vi "Kickforce.vi"(8 "AI Parameters":T1={"GotoKick"={"Dist do cone a frente"=150.0, "attacker farback"=1500.0, "Perto"=300.0, "min dist to kick"=150.0, "kick eps"=0.05, "Time to transition"=0.0}, "Attacker"={"CC chute"=0.09, "CC passe"=0.045, "Kick Force"=100.0, "ball-robot Kick"=200.0, "ball-robot Pass"=0.3, "drible\nAttk"=FALSE}, "Defender"={"D max"=1700.0, "Vel p/ robô av"=1000.0, "Kick Force"=100.0, "D atk-def"=0.0, "D farback"=0.0, "drible\ndef"=FALSE, "drible\ngoalie"=FALSE}, "Timeout"={"Field/v in x"=6.0, "Dist Robots"=300, "Dist up in y"=300}, "Pose Striker"={"dist"=200.0, "Numeric"=-4.0, "dist 2"=200.0, "drible\nstriker"=FALSE}, "Dist Stop"=300.0, "D ball out"=200, "D central gap "=150.0, "T pass"=0.0, "Force ++"=0.0, "range kick"=0.0, "Chute alto"=TRUE, "Marcador novo"=TRUE, "drible"=FALSE, "D drible"=300.0} {"D drible" format="%#_13g"; "D central gap" format="%#_13g"; "Dist Stop" format="%#_13g"; "Pose Striker"."Numeric" format="%#_13g"; "Defender"."Kick Force" format="%#_13g"; "Defender"."Vel p/ robô av" format="%#_13g"; "Attacker"."ball-robot Kick" format="%#_13g"; "Attacker"."Kick Force" format="%#_13g"; "Attacker"."CC passe" format="%#_13g"; "Attacker"."CC chute" format="%#_13g"; "GotoKick"."kick eps" format="%#_13g"; "GotoKick"."min dist to kick" format="%#_13g"; "GotoKick"."Perto" format="%#_13g"; "GotoKick"."attacker farback" format="%#_13g"; "GotoKick"."Dist do cone a frente" format="%#_13g"}, 10 "Distância ao\nalvo do chute":dbl=1.23 format="%#_13g") -> (1 "Tempo até  bola\nchegar ao alvo":dbl, 2 "Força do chute":dbl)   [LabVIEW 2017]
uses:
  AI Parameters.ctl
panel:
  in  "y":dbl=12.0
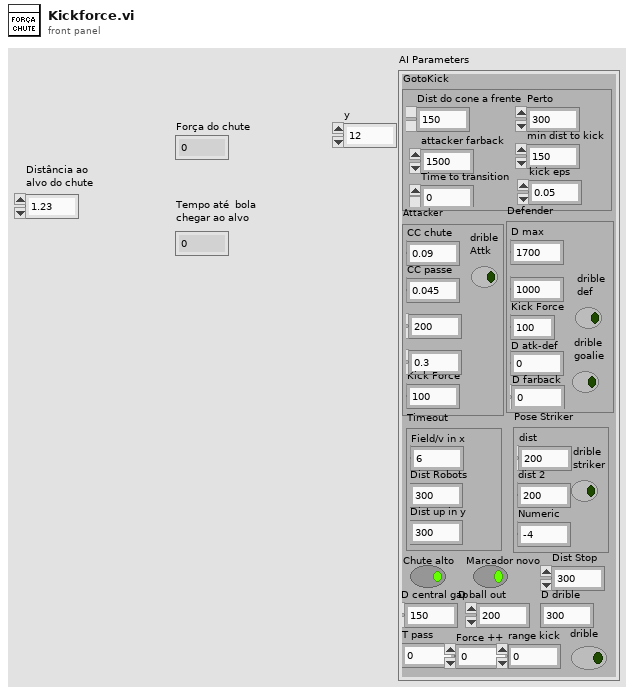
[diagram p1: front panel]
types:
  T1 = typedef "AI Parameters.ctl" = cluster{"GotoKick":cluster{"Dist do cone a frente":dbl, "attacker farback":dbl, "Perto":dbl, "min dist to kick":dbl, "kick eps":dbl, "Time to transition":dbl}, "Attacker":cluster{"CC chute":dbl, "CC passe":dbl, "Kick Force":dbl, "ball-robot Kick":dbl, "ball-robot Pass":dbl, "drible\nAttk":bool}, "Defender":cluster{"D max":dbl, "Vel p/ robô av":dbl, "Kick Force":dbl, "D atk-def":dbl, "D farback":dbl, "drible\ndef":bool, "drible\ngoalie":bool}, "Timeout":cluster{"Field/v in x":dbl, "Dist Robots":u32, "Dist up in y":u32}, "Pose Striker":cluster{"dist":dbl, "Numeric":dbl, "dist 2":dbl, "drible\nstriker":bool}, "Dist Stop":dbl, "D ball out":i32, "D central gap ":dbl, "T pass":dbl, "Force ++":dbl, "range kick":dbl, "Chute alto":bool, "Marcador novo":bool, "drible":bool, "D drible":dbl}
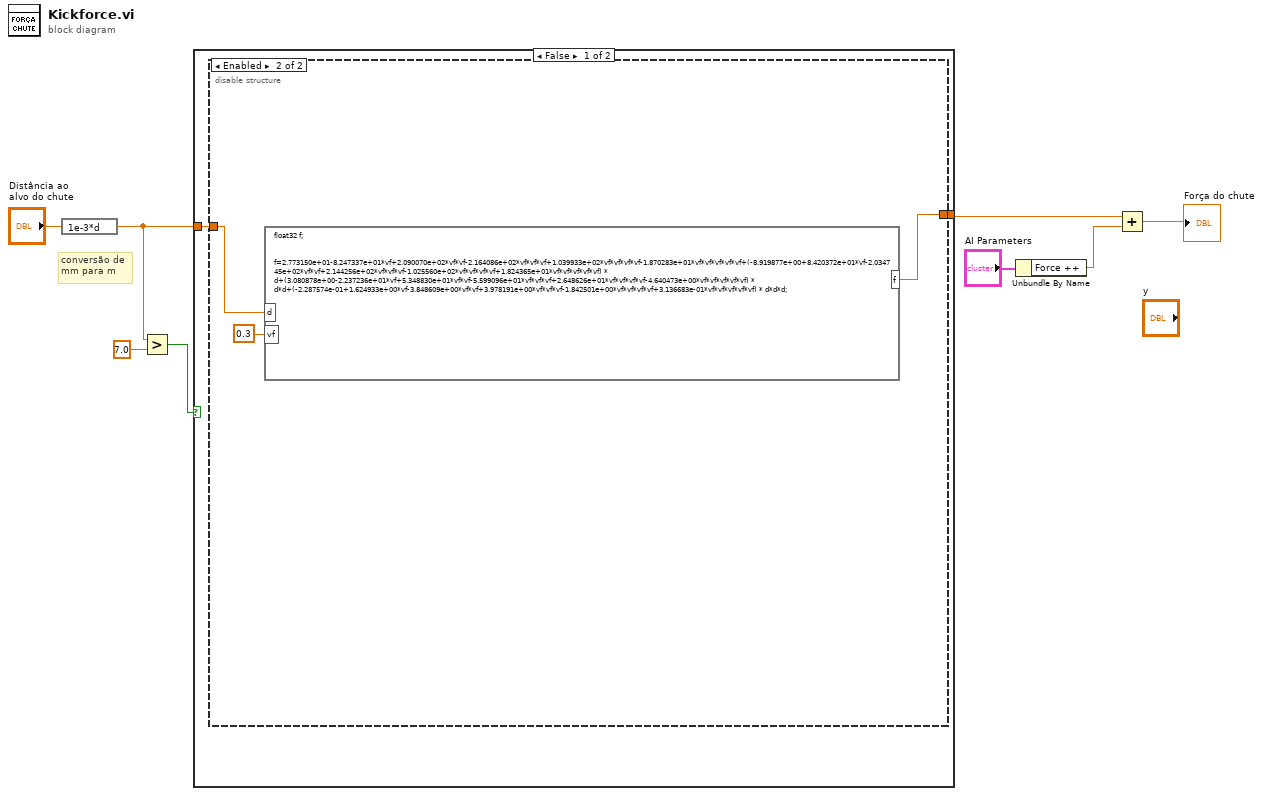
[diagram p0: block diagram]
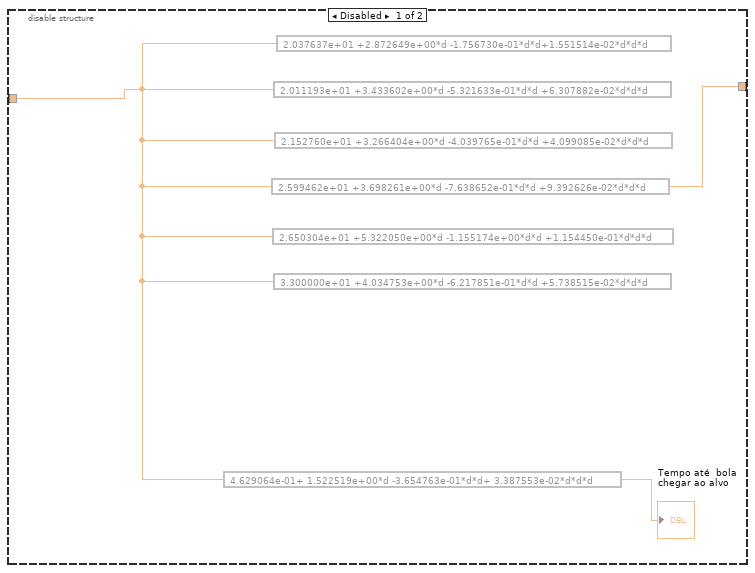
[diagram p2: hidden frame]
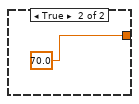
[diagram p3: hidden frame]
diagram:
  # "conversão de\nmm para m"
  n1 = expression code="1e-3*d"("Distância ao\nalvo do chute") -> (w5:dbl)
  n2 = Greater?(x=w5, y=7.0) -> (0:w3:bool)
  n3 = case shown="False" w3 {
    tunnel: w5 -> [w10 _]
    tunnel: [w9 70.0] -> w6
    frame False {
      n4 = disable-structure shown="Enabled" {
        disable-tunnel: w10 -> [w13 w16]
        disable-tunnel: [w11 w15] -> w9
        frame Disabled {
          n5 = expression code="4.629064e-01+ 1.522519e+00*d -3.654763e-01*d*d+ 3.387553e-02*d*d*d"(w13) -> (→"Tempo até  bola\nchegar ao alvo":dbl)
          n6 = expression code="2.599462e+01 +3.698261e+00*d -7.638652e-01*d*d +9.392626e-02*d*d*d"(w13) -> (w11:dbl)
          n7 = expression code="2.650304e+01 +5.322050e+00*d -1.155174e+00*d*d +1.154450e-01*d*d*d"(w13) -> ()  [unwired: 1 out]
          n8 = expression code="2.011193e+01 +3.433602e+00*d -5.321633e-01*d*d +6.307882e-02*d*d*d"(w13) -> ()  [unwired: 1 out]
          n9 = expression code="3.300000e+01 +4.034753e+00*d -6.217851e-01*d*d +5.738515e-02*d*d*d"(w13) -> ()  [unwired: 1 out]
          n10 = expression code="2.152760e+01 +3.266404e+00*d -4.039765e-01*d*d +4.099085e-02*d*d*d"(w13) -> ()  [unwired: 1 out]
          n11 = expression code="2.037637e+01 +2.872649e+00*d -1.756730e-01*d*d+1.551514e-02*d*d*d"(w13) -> ()  [unwired: 1 out]
        }
        frame Enabled {
          n12 = formula code="float32 f;\n\n\nf=2.773150e+01-8.247337e+01*vf+2.090070e+02*vf*vf-2.164086e+02*vf*vf*vf+1.039933e+02*vf*vf*vf*vf-1.870283e+01*vf*vf*vf*vf*vf+(-8.919877e+00+8.420372e+01*vf-2.034745e+02*vf*vf+2.144256e+02*vf*vf*vf-1.025560e+02*vf*vf*vf*vf+1.824365e+01*vf*vf*vf*vf*vf) * d+(3.080878e+00-2.237236e+01*vf+5.348830e+01*vf*vf-5.599096e+01*vf*vf*vf+2.648626e+01*vf*vf*vf*vf-4.640473e+00*vf*vf*vf*vf*vf) * d*d+(-2.287574e-01+1.624933e+00*vf-3.848609e+00*vf*vf+3.978191e+00*vf*vf*vf-1.842501e+00*vf*vf*vf*vf+3.136683e-01*vf*vf*vf*vf*vf) * d*d*d;"("d"=w16, "vf"=0.3 ("input variable")) -> ("f"=w15:sgl)
        }
      }
    }
    frame True {
    }
  }
  n13 = Unbundle By Name("AI Parameters") -> ("Force ++"=w1:dbl)
  n14 = Add(x=w6, y=w1) -> (x+y=→"Força do chute":dbl)
